vi "SECoP_dataGetMinMaxInteger.vi"(7 "Position":u32, 8 "error in (no error)":errorcluster, 10 "SECoP_dataPtr":T1 {"ptr64" format="%.0x"; "ptr32" format="%.0x"}, 11 "DLL path (in)":T2) -> (0 "error out":errorcluster, 1 "maximum value":i64, 2 "minimum value":i64, 3 "DLL path (out)":T2)   [LabVIEW 2023, in "SECoP.lvlib"]
doc: "Call <b>\"SECoP_dataGetMinMaxInteger.vi\"</b> to access the minimum and maximum value (integer or scaled of SECoP_dataPtr).\n\n<b>DLL path</b> input and output of cluster from \"SECoP-Initialize.vi\"\n<b>SECoP_dataPtr</b> data to access\n<b>Position</b> points to a virtual flattened entry of the data type\n<b>minimum value</b> minimal allowed numeric/unscaled value\n<b>maximum value</b> maximal allowed numeric/unscaled value"
uses:
  SECoP.lvlib
  SECoP-libraries.ctl
  SECoP-data.ctl
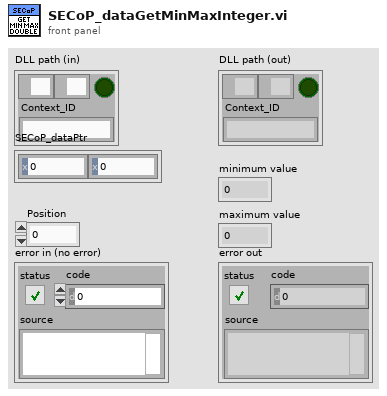
[diagram p1: front panel]
types:
  T1 = typedef "SECoP.lvlib/SECoP-data.ctl" = cluster{"ptr32":u32, "ptr64":u64}
  T2 = typedef "SECoP.lvlib/SECoP-libraries.ctl" = cluster{"serverDLL":path, "variantDLL":path, "cleanup_mode":bool, "Context_ID":string}
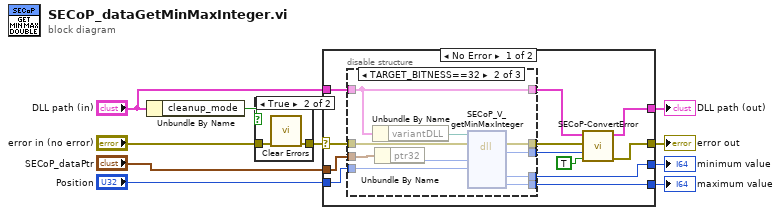
[diagram p0: block diagram]
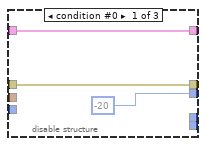
[diagram p3: hidden frame]
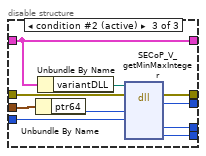
[diagram p4: hidden frame]
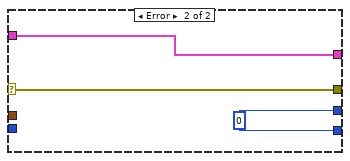
[diagram p5: hidden frame]
diagram:
  n1 = Unbundle By Name("DLL path (in)") -> ("cleanup_mode"=w7:bool)
  n2 = case shown="True" w7 {
    tunnel: "error in (no error)" -> [w11 w13]
    tunnel: [w11 w12] -> w5
    frame False {
    }
    frame True {
      n3 = call <vilib>:"Clear Errors.vi"("error in (no error)"=w13) -> ("error out"=w12:errorcluster)  [unwired: 5 in, 1 out]
    }
  }
  n4 = case shown="No Error" w5 {
    selector: w5 -> [w24 w50]
    tunnel: "DLL path (in)" -> [w23 w51]
    tunnel: [w14 w51] -> w9
    tunnel: [w25 w50] -> w8
    tunnel: "Position" -> [w19 _]
    tunnel: [w18 w49] -> w3
    tunnel: "SECoP_dataPtr" -> [w17 _]
    tunnel: [w16 w49] -> w1
    frame No Error {
      n5 = disable-structure shown="TARGET_BITNESS==32" {
        disable-tunnel: w24 -> [w28 w38 w48]
        disable-tunnel: w23 -> [w26 w30 w40]
        disable-tunnel: [w28 w37 w47] -> w22
        disable-tunnel: [-20 w36 w46] -> w21
        disable-tunnel: w19 -> [_ w35 w45]
        disable-tunnel: [_ w34 w44] -> w18
        disable-tunnel: w17 -> [_ w32 w42]
        disable-tunnel: [_ w31 w41] -> w16
        disable-tunnel: [w26 w30 w40] -> w15
        frame condition #0 {
        }
        frame condition #1 {
          n6 = Unbundle By Name(w30) -> ("variantDLL"=w29:path)
          n7 = Unbundle By Name(w32) -> ("ptr32"=w33:u32)
          n8 = dll-call lib="Z:/Praktische_Aufgaben/SECoP-LabVIEW2015/32bit/SECoP32.dll" fn="SECoP_V_getMinMaxInteger"(path in=w29, error in=w38, "pData"=w33, "uPosition"=w35) -> (error out=w37:errorcluster, "return type"=w36:i32, "llMinimum"=w31:i64, "llMaximum"=w34:i64)  [unwired: 5 in, 1 out]
        }
        frame condition #2 (active) {
          n9 = Unbundle By Name(w42) -> ("ptr64"=w43:u64)
          n10 = Unbundle By Name(w40) -> ("variantDLL"=w39:path)
          n11 = dll-call lib="Z:/Praktische_Aufgaben/SECoP-LabVIEW2015/32bit/SECoP32.dll" fn="SECoP_V_getMinMaxInteger"(path in=w39, error in=w48, "pData"=w43, "uPosition"=w45) -> (error out=w47:errorcluster, "return type"=w46:i32, "llMinimum"=w41:i64, "llMaximum"=w44:i64)  [unwired: 5 in, 1 out]
        }
      }
      n12 = call "SECoP-ConvertError.vi"("return is boolean"=TRUE, "return code"=w21, "error in (no error)"=w22, "DLL path (in)"=w15) -> ("error out"=w25:errorcluster, "DLL path (out)"=w14:T2)  [unwired: 6 in]
    }
    frame Error {
      w49 = i64 0 ("Value")
    }
  }
  "DLL path (out)" <- w9
  "error out" <- w8
  "maximum value" <- w3
  "minimum value" <- w1
